vi "HEWH Check UE Cutout For Condition Change.vi"(4 "Check For New  Condition":bool, 7 "HEWH Specific DAQ":T8, 9 "Current Sequence Index":i32, 10 "Terminate Condition in":T3, 11 "PRAT/RLT Sequence":T1[](array[typedef]) {"Time" format="%<%H:%M:%S>t"}) -> (2 "Terminate Condition out":T3, 3 "PRAT/RLT Sequence (Output)":T1[](array[typedef]) {"Time" format="%<%H:%M:%S>t"})   [LabVIEW 2016]
uses:
  Type Definitions/HEWH Specific DAQ.ctl
  Type Definitions/HEWH Power Data.ctl
  Type Definitions/HEWH Power Elements.ctl
  Utility/Type Definitions/UTILITY Power Analyzer.ctl
  Draw Water Specific/Type Definitions/Terminate Draw Conditions.ctl
  Type Definitions/PRAT Test.ctl
  Utility/Save File/File Setup (Public)/Type Definition/Save File HEWH Heating Control Mode.ctl
  Type Definitions/HEWH Start Conditions.ctl
  Draw Water Specific/Type Definitions/Check Special Condtions.ctl
  Draw Water Specific/Type Definitions/HEWH Special Condition Check.ctl
  Type Definitions/HEWH Draw Flag ENUM.ctl
  Utility/Save File/File Setup.lvlib
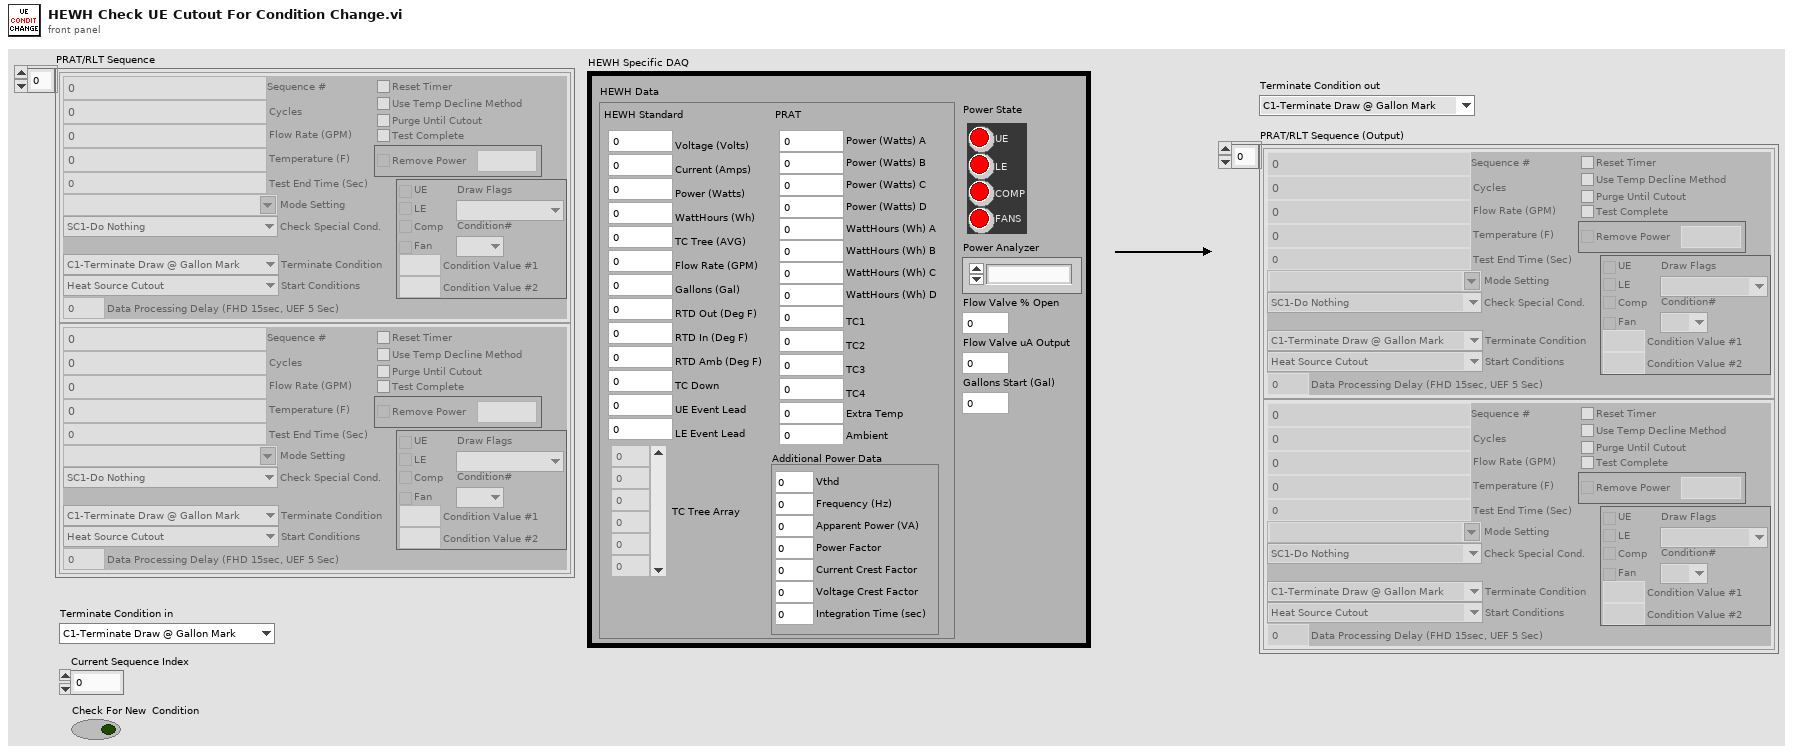
[diagram p1: front panel]
types:
  T1 = typedef "PRAT Test.ctl" = cluster{"Sequence #":dbl, "Cycles":i32, "Mode Setting":T2, "Flow Rate (GPM)":dbl, "Temperature (F)":dbl, "Reset Timer":bool, "Use Temp Decline Method":bool, "Terminate Condition":T3, "Condition Value #1":dbl, "UE":bool, "LE":bool, "Comp":bool, "Fan":bool, "Test End Time (Sec)":dbl, "Purge Until Cutout":bool, "Start Conditions":T4, "Condition Value #2":dbl, "Remove Power":bool, "Time":dbl, "Check Special Cond.":T5, "Condition#":T6, "Draw Flags":T7, "Data Processing Delay (FHD 15sec, UEF 5 Sec)":dbl, "Test Complete":bool}
  T2 = typedef "File Setup.lvlib/Save File HEWH Heating Control Mode.ctl" = string
  T3 = typedef "Terminate Draw Conditions.ctl" = enum16{"C1-Terminate Draw @ Gallon Mark", "C2-Special Last Draw (HU Test)", "C3-RTD Out <=", "C4-Mean Tank Temp <=", "C5-Decrease RTD Out (Deg F)", "C6-Time (Seconds)", "C7-Until Any Heat Source", "C8-Specific Heat Source", "C9-Do Nothing"}
  T4 = typedef "HEWH Start Conditions.ctl" = enum16{"Heat Source Cutout", "At Time (Seconds)", "Every X (Seconds)", "T2 >= X° Below Setpoint", "Seconds From Complete", "Wait for LE & Comp Cutout", "Wait for Comp Cutout", "Wait for LE Cutout", "Wait for UE Cutout"}
  T5 = typedef "Check Special Condtions.ctl" = enum16{"SC1-Do Nothing", "SC2-Check Heat Source (On-C2/Off-C1)", "SC3-Check Skip Condition", "SC4-Check Heat Source ON/Fail"}
  T6 = typedef "HEWH Special Condition Check.ctl" = enum16{"N/A", "C1", "C2", "Reset/Fail", "Skip Draw Sequence"}
  T7 = typedef "HEWH Draw Flag ENUM.ctl" = enum16{"N/A", "None(0)", "Sml(1)", "Med(2)", "SmlMed(3)", "Lrg(4)", "SmlLrg(5)", "MedLrg(6)", "SmlMedLrg(7)"}
  T8 = typedef "HEWH Specific DAQ.ctl" = cluster{"HEWH Data":T9, "Flow Valve % Open":dbl, "Power State":T10, "Power Analyzer":T11, "Flow Valve uA Output":i32, "Gallons Start (Gal)":dbl}
  T9 = typedef "HEWH Power Data.ctl" = cluster{"HEWH Standard":cluster{"Voltage (Volts)":dbl, "Current (Amps)":dbl, "Power (Watts)":dbl, "WattHours (Wh)":dbl, "TC Tree (AVG)":dbl, "Flow Rate (GPM)":dbl, "Gallons (Gal)":dbl, "RTD Out (Deg F)":dbl, "RTD In (Deg F)":dbl, "RTD Amb (Deg F)":dbl, "TC Down":dbl, "UE Event Lead":i32, "LE Event Lead":i32, "TC Tree Array":dbl[]}, "PRAT":cluster{"Power (Watts) A":dbl, "Power (Watts) B":dbl, "Power (Watts) C":dbl, "Power (Watts) D":dbl, "TC1":dbl, "TC2":dbl, "TC3":dbl, "TC4":dbl, "WattHours (Wh) A":dbl, "WattHours (Wh) B":dbl, "WattHours (Wh) C":dbl, "WattHours (Wh) D":dbl, "Ambient":dbl, "Extra Temp":dbl}, "Additional Power Data":cluster{"Vthd":dbl, "Frequency (Hz)":dbl, "Apparent Power (VA)":dbl, "Power Factor":dbl, "Current Crest Factor":dbl, "Voltage Crest Factor":dbl, "Integration Time (sec)":dbl}}
  T10 = typedef "HEWH Power Elements.ctl" = cluster{"UE":bool, "LE":bool, "COMP":bool, "FANS":bool}
  T11 = typedef "UTILITY Power Analyzer.ctl" = enum16{"", "APLUS", "WT210", "WT500", "WT300", "OSI", "Debug", "WT230", "WT300_1", "WT300_2"}
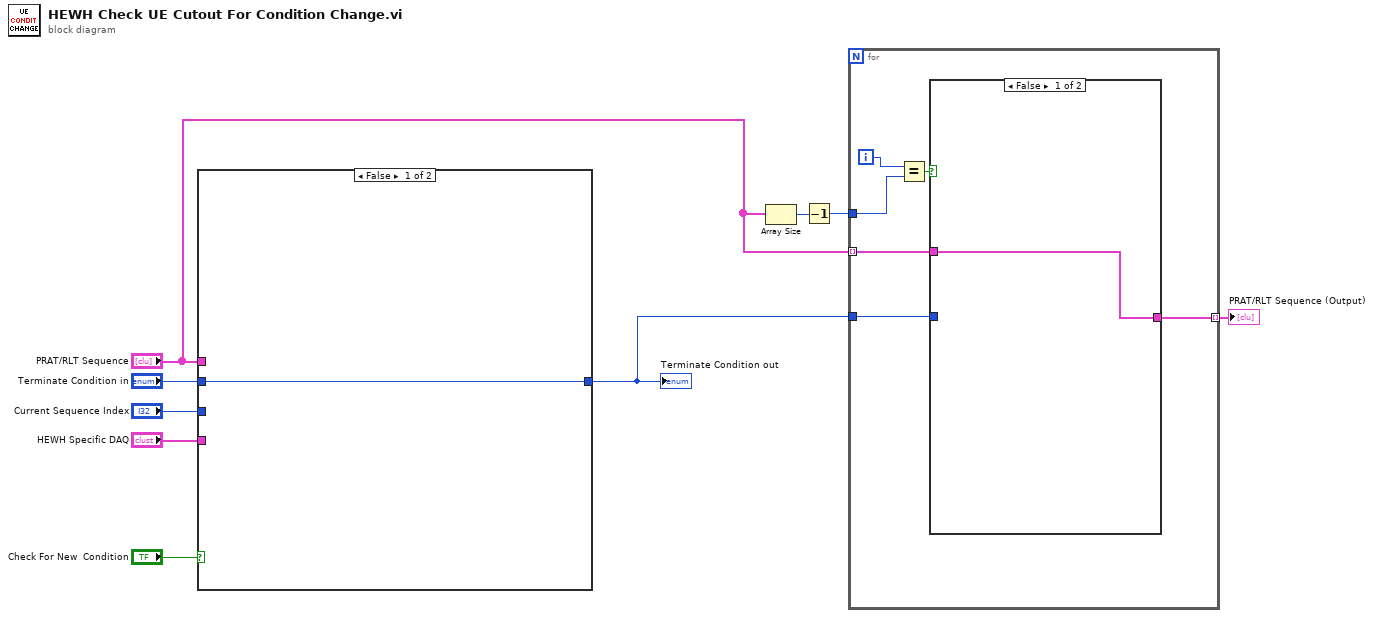
[diagram p0: block diagram]
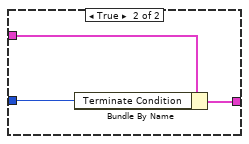
[diagram p2: hidden frame]
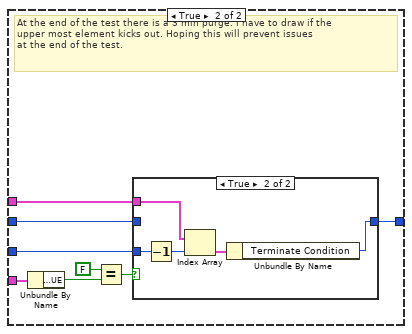
[diagram p3: hidden frame]
diagram:
  n1 = case shown="False" "Check For New  Condition" {
    tunnel: "HEWH Specific DAQ" -> [_ w16]
    tunnel: "Terminate Condition in" -> [w10 w14]
    tunnel: [w10 w13] -> w2
    tunnel: "PRAT/RLT Sequence" -> [_ w12]
    tunnel: "Current Sequence Index" -> [_ w11]
    frame False {
    }
    frame True {
      # "At the end of the test there is a 3 min purge. I have to draw if the\nupper most element kicks out. Hoping this will prevent issues \nat the end of the test."
      n2 = Unbundle By Name(w16) -> ("Power State.UE"=w17:bool)
      n3 = Equal?(x=FALSE, y=w17) -> (x = y?=w15:bool)
      n4 = case shown="True" w15 {
        tunnel: w14 -> [w19 _]
        tunnel: [w19 w21] -> w13
        tunnel: w12 -> [_ w24]
        tunnel: w11 -> [_ w23]
        frame False {
        }
        frame True {
          n5 = Decrement(x=w23) -> (x-1=w20:i32)
          n6 = Index Array(array=w24, index=w20) -> (element=w22:T1)
          n7 = Unbundle By Name(w22) -> ("Terminate Condition"=w21:T3)
        }
      }
    }
  }
  "Terminate Condition out" <- w2
  n8 = Array Size(array="PRAT/RLT Sequence") -> (size(s)=w4:i32)
  n9 = Decrement(x=w4) -> (x-1=w3:i32)
  n10 = for {
    tunnel: "PRAT/RLT Sequence" -> [w27] mode=indexing
    tunnel: w3 -> [w30]
    tunnel: [w26] -> w1 mode=indexing
    tunnel: w2 -> [w25]
    i -> [w29]
    n11 = Equal?(x=w29, y=w30) -> (x = y?=w28:bool)
    n12 = case shown="False" w28 {
      tunnel: w27 -> [w31 w34]
      tunnel: [w31 w33] -> w26
      tunnel: w25 -> [_ w32]
      frame False {
      }
      frame True {
        n13 = Bundle By Name(cluster=w34, "Terminate Condition"=w32) -> (w33:T1)
      }
    }
  }
  "PRAT/RLT Sequence (Output)" <- w1
